vi "Handle Last Ack Core.vi"(4 "error in (no error)":errorcluster, 6 "Last Ack":refnum<class "Last Ack.lvclass">, 7 "MVVM Abstruct View in":refnum<class "MVVM Abstruct View.lvclass">) -> (0 "error out":errorcluster, 3 "MVVM Abstruct View out":refnum<class "MVVM Abstruct View.lvclass">)   [LabVIEW 2020, in "MMVVM Framework.lvlib" / "MVVM Abstruct View.lvlib" / "MVVM Abstruct View.lvclass"]
doc: "(<B>Filename</B>: Actor Framework.lvlib:Actor.lvclass:Handle Last Ack Core.vi)\n\nDefines how the caller actor responds to the Last Ack message from a nested actor. The Last Ack message is the final message a nested actor sends to its caller before it shuts down. The message contains information about the final state of the nested actor.\n\nBy default, this method does nothing except return any error the nested actor sent. A descendant class may override this method to define behavior."
uses:
  MVVM Abstruct View.lvclass
  <vilib>/ActorFramework/LastAck/Last Ack.lvclass
  <vilib>/ActorFramework/LastAck/Last Ack.lvclass/Last Ack.ctl
  Abstruct View/Abstruct View/Abstruct View.lvclass
  <vilib>/ActorFramework/Actor/Actor.lvclass
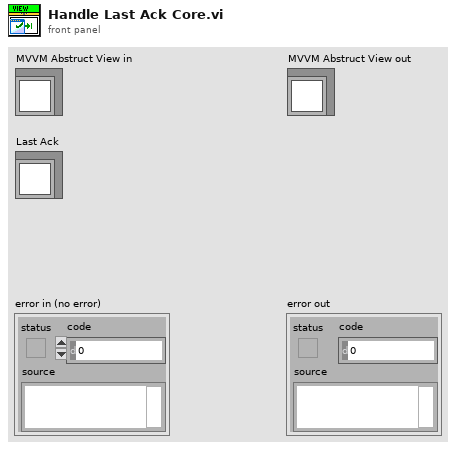
[diagram p1: front panel]
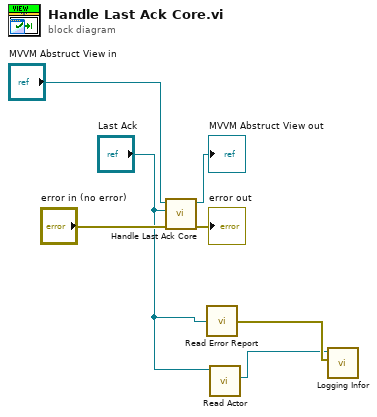
[diagram p0: block diagram]
diagram:
  n1 = call-parent "Handle Last Ack Core.vi"("error in (no error)"="error in (no error)", "Last Ack"="Last Ack", "Actor in"="MVVM Abstruct View in") -> ("error out"=→"error out":errorcluster, "Actor out"=→"MVVM Abstruct View out":refnum<class "MVVM Abstruct View.lvclass">)  [unwired: 3 in]
  n2 = call <vilib>:"Read Error Report.vi"("Last Ack"="Last Ack") -> ("error report"=w2:errorcluster)
  n3 = call <vilib>:"Read Actor.vi"("Last Ack"="Last Ack") -> ("Actor"=w1:refnum<class "Actor.lvclass">)  [unwired: 10 in]
  n4 = call "Logging Infor.vi"("error in (no error)"=w2, "Class"=w1) -> ()  [unwired: 9 in, 1 out]
